vi "Init Main Panels.vi"(8 "error in (no error)":errorcluster, 11 "App in":refnum<class "App.lvclass">) -> (0 "error out":errorcluster, 3 "App out":refnum<class "App.lvclass">)   [LabVIEW 2020, in "PicoG-App.lvlib" / "App.lvclass"]
uses:
  App.lvclass
  GettingStarted/GettingStarted.lvclass
  C:/Program Files (x86)/National Instruments/LabVIEW 2020/vi.lib/IlluminatedG/IG OOPanel/OOPanel/Panel/Panel.lvclass
  AppDetailPanel/AppDetailPanel.lvclass
  PlatformConfigPanel/PlatformConfigPanel.lvclass
  DeviceDetailPanel/DeviceDetailPanel.lvclass
  App.lvclass/App.ctl
  <vilib>/IlluminatedG/IG OOPanel/OOPanel/Manager/Manager.lvclass
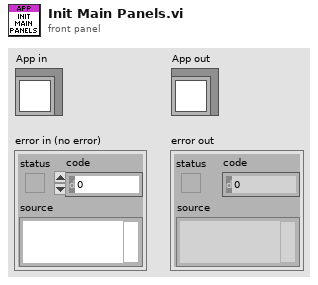
[diagram p1: front panel]
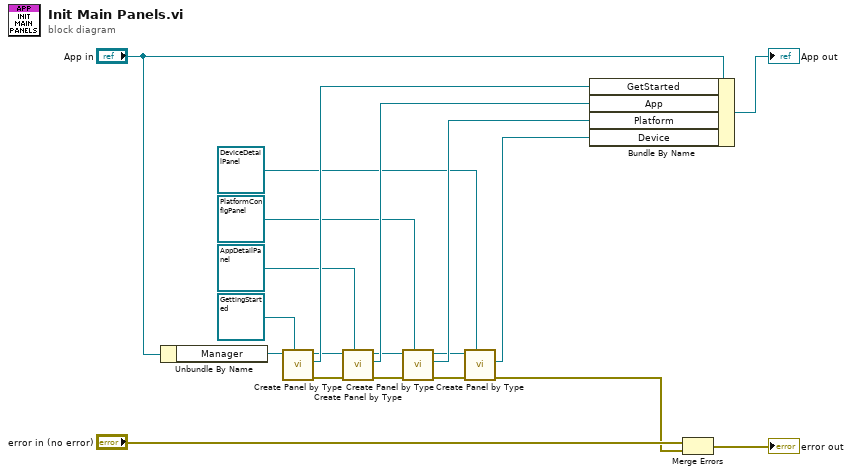
[diagram p0: block diagram]
diagram:
  n1 = Unbundle By Name("App in") -> ("Manager"=w17:refnum<class "Manager.lvclass">)
  n2 = call <vilib>:"Create Panel by Type.vi"("Panel Type"=refnum<class "GettingStarted.lvclass"> refnum ("PicoG-App.lvlib:GettingStarted.lvclass"), "Manager in"=w17) -> ("error out"=w11:errorcluster, "Panel"=w15:refnum<class "GettingStarted.lvclass">, "Manager out"=w14:refnum<class "Manager.lvclass">)  [unwired: 7 in]
  n3 = call <vilib>:"Create Panel by Type.vi"("Panel Type"=refnum<class "AppDetailPanel.lvclass"> refnum ("PicoG-App.lvlib:AppDetailPanel.lvclass"), "error in (no error)"=w11, "Manager in"=w14) -> ("error out"=w9:errorcluster, "Panel"=w12:refnum<class "AppDetailPanel.lvclass">, "Manager out"=w8:refnum<class "Manager.lvclass">)  [unwired: 6 in]
  n4 = call <vilib>:"Create Panel by Type.vi"("Panel Type"=refnum<class "PlatformConfigPanel.lvclass"> refnum ("PicoG-App.lvlib:PlatformConfigPanel.lvclass"), "error in (no error)"=w9, "Manager in"=w8) -> ("error out"=w4:errorcluster, "Panel"=w6:refnum<class "PlatformConfigPanel.lvclass">, "Manager out"=w5:refnum<class "Manager.lvclass">)  [unwired: 6 in]
  n5 = call <vilib>:"Create Panel by Type.vi"("Panel Type"=refnum<class "DeviceDetailPanel.lvclass"> refnum ("PicoG-App.lvlib:DeviceDetailPanel.lvclass"), "error in (no error)"=w4, "Manager in"=w5) -> ("error out"=w2:errorcluster, "Panel"=w1:refnum<class "DeviceDetailPanel.lvclass">)  [unwired: 6 in, 1 out]
  n6 = Bundle By Name(cluster="App in", "GetStarted"=w15, "App"=w12, "Platform"=w6, "Device"=w1) -> (→"App out":refnum<class "App.lvclass">)
  n7 = Merge Errors("error in (no error)", w2) -> (→"error out":errorcluster)
